vi "ExerciceSerrure.vi"() -> ()   [LabVIEW 2018]
panel:
  out "LED":bool
  in  "Cadenas 3":i8(knob) scale=0.0..9.0
  in  "Cadenas  2":i8(knob) scale=0.0..9.0
  in  "Cadenas 1":i8(knob) scale=0.0..9.0
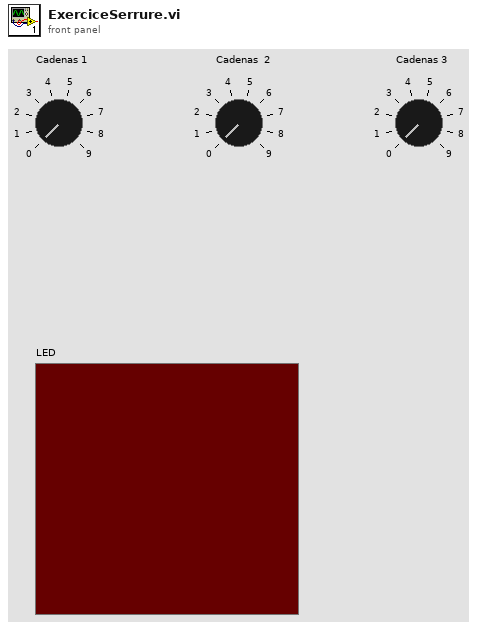
[diagram p1: front panel]
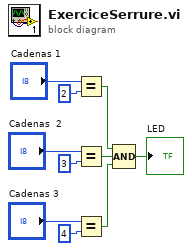
[diagram p0: block diagram]
diagram:
  n1 = Equal?(x="Cadenas 1", y=i8 2) -> (x = y?=w4:bool)
  n2 = Equal?(x="Cadenas  2", y=i8 3) -> (x = y?=w3:bool)
  n3 = Equal?(x="Cadenas 3", y=i8 4) -> (x = y?=w2:bool)
  n4 = Compound Arithmetic op=AND(w4, w3, w2) -> (→"LED":bool)
